vi "FGV-GEvt Filter Obj.vi"(6 "Set(T)/Get(F)":bool, 8 "Error in":errorcluster caption="Error in (no error)", 11 "Rules-v1":T1) -> (0 "Error out":errorcluster, 3 "CSM:LogFilter.lvclass":refnum<class "LogFilter.lvclass">)   [LabVIEW 2020, in "Communicable State Machine.lvlib"]
uses:
  Communicable State Machine.lvlib
  LogFilter.lvclass
  _CSM_GlobalLog Filter Rules - v1.0.ctl
  _CSM_GlobalLog_MSG_TYPE.ctl
  _CSM_GlobalLog_STATE_TYPE.ctl
  global-GEvnt Filter Change Flag.vi
  Set Global CSM Filter.vi
  Set Global LogType Filter.vi
  Set Global State Filter.vi
  Set CSM LogType Filter.vi
  Set CSM State Filter.vi
  Set Global StateType Filter.vi
  Set CSM StateType Filter.vi
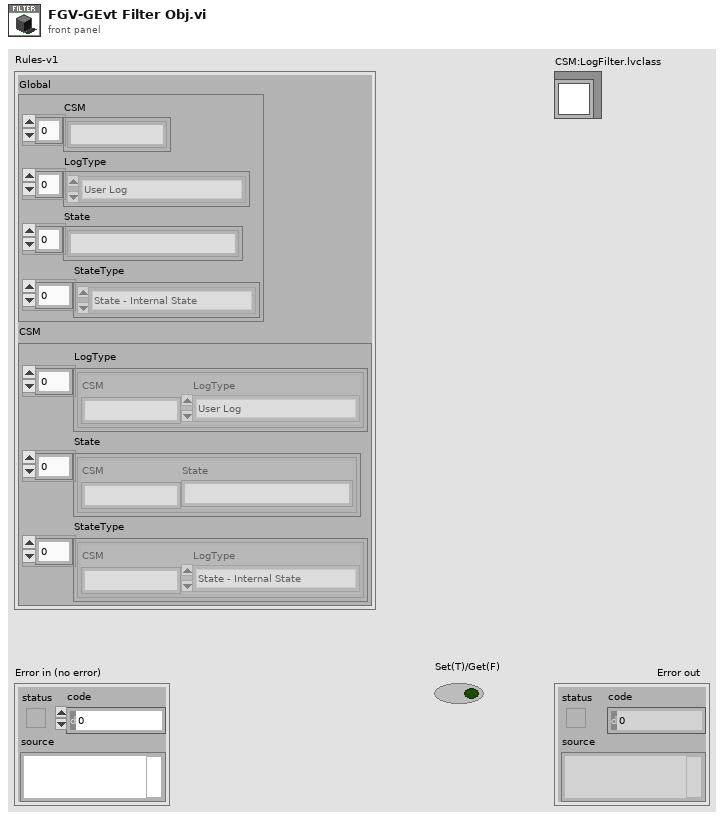
[diagram p1: front panel]
types:
  T1 = typedef "Communicable State Machine.lvlib/_CSM_GlobalLog Filter Rules - v1.0.ctl" = cluster{"Global":cluster{"CSM":string[], "LogType":T2[], "State":string[], "StateType":T3[]}, "CSM":cluster{"LogType":cluster{"CSM":string, "LogType":T2}[], "State":cluster{"CSM":string, "State":string}[], "StateType":cluster{"CSM":string, "LogType":T3}[]}}
  T2 = typedef "Communicable State Machine.lvlib/_CSM_GlobalLog_MSG_TYPE.ctl" = enum16{"User Log", "State Change", "Status", "Interrupt", "Register", "Unregister", "Error Log", "Module Created", "Module Destroyed"}
  T3 = typedef "Communicable State Machine.lvlib/_CSM_GlobalLog_STATE_TYPE.ctl" = enum16{"State - Internal State", "State - External Message", "State - Response", "State - Complete"}
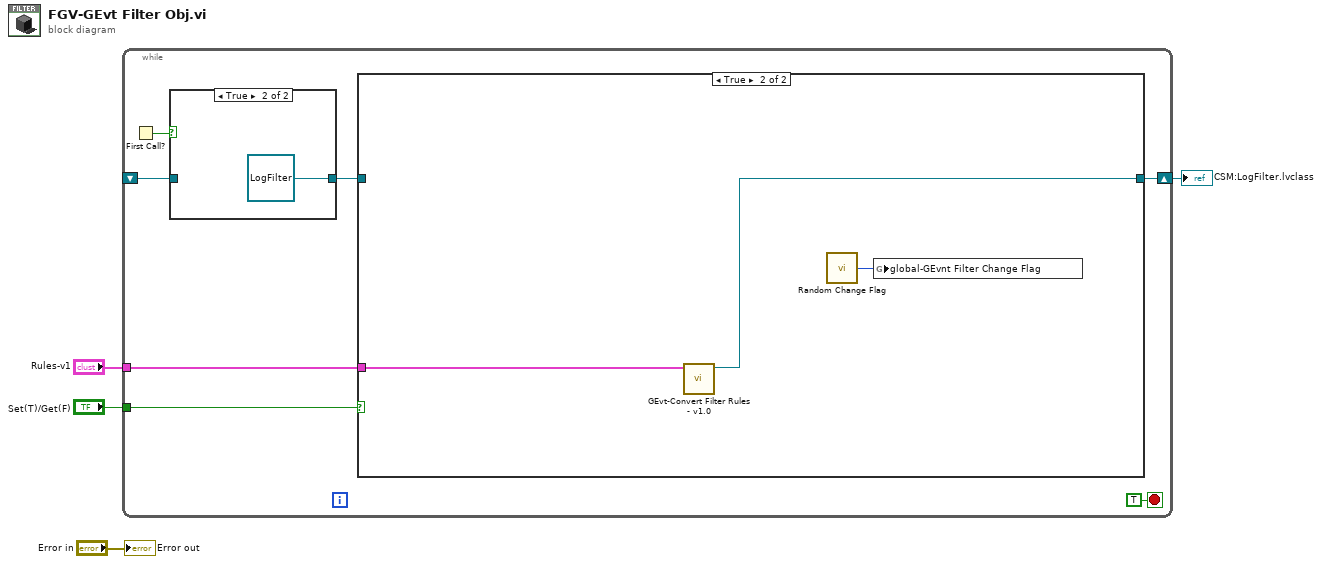
[diagram p0: block diagram]
diagram:
  n1 = while {
    shift-right: [w8] -> w3
    shift-left: _ -> [w7]
    tunnel: "Set(T)/Get(F)" -> [w6]
    tunnel: "Rules-v1" -> [w5]
    stop <- TRUE stop-if-true
    n2 = First Call?() -> (First Call?: T/F=w10:bool)
    n3 = case shown="True" w10 {
      tunnel: [w12 refnum<class "LogFilter.lvclass"> refnum ("CSM:LogFilter.lvclass")] -> w9
      tunnel: w7 -> [w12 _]
      frame False {
      }
      frame True {
      }
    }
    n4 = case shown="True" w6 {
      tunnel: w9 -> [w14 _]
      tunnel: [w14 w17] -> w8
      tunnel: w5 -> [_ w16]
      frame False {
      }
      frame True {
        n5 = call "GEvt-Convert Filter Rules - v1.0.vi"("Rules-v1"=w16) -> ("GlobalLogFilter"=w17:refnum<class "LogFilter.lvclass">)  [unwired: 10 in]
        n6 = call "Random Change Flag.vi"() -> ("Random Change Flag"=w15:u64)  [unwired: 2 in]
        n7 = global write "global-GEvnt Filter Change Flag.vi" "global-GEvnt Filter Change Flag"(w15) -> ()
      }
    }
  }
  "CSM:LogFilter.lvclass" <- w3
  "Error out" <- "Error in"
